vi "Multiserver Example.vi"() -> ()   [LabVIEW 2013]
uses:
  LabVIEW Core/Ports - Keep-Alive, LabVIEW-to-Python, Python-to-LabVIEW.ctl
  LabVIEW Core/TS.lvlib
panel:
  in  "Local IP Address for LabVIEW Server 2":string="localhost"
  in  "Ports 2":T1={"KA Port (9007)"=9010, "LtoP Port (9008)"=9011, "PtoL Port (9009)"=9012}
  in  "Server Alias 2":string="Test Group 2"
  in  "Local IP Address for LabVIEW Server 1":string="localhost"
  in  "Ports 1":T1={"KA Port (9007)"=9007, "LtoP Port (9008)"=9008, "PtoL Port (9009)"=9009}
  in  "Server Alias 1":string="Test Group 1"
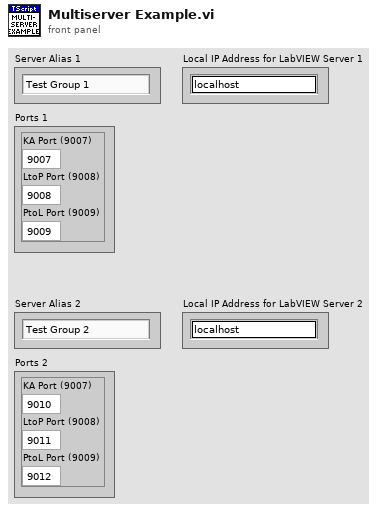
[diagram p1: front panel]
types:
  T1 = typedef "TS.lvlib/Ports - Keep-Alive, LabVIEW-to-Python, Python-to-LabVIEW.ctl" = cluster{"KA Port (9007)":u16, "LtoP Port (9008)":u16, "PtoL Port (9009)":u16}
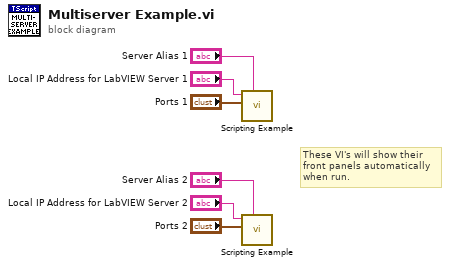
[diagram p0: block diagram]
diagram:
  # "These VI's will show their\nfront panels automatically \nwhen run."
  n1 = call "Scripting Example.vi"("Server Alias"="Server Alias 1", "Ports"="Ports 1", "Local IP Address for LabVIEW Server"="Local IP Address for LabVIEW Server 1") -> ()  [unwired: 9 in]
  n2 = call "Scripting Example.vi"("Server Alias"="Server Alias 2", "Ports"="Ports 2", "Local IP Address for LabVIEW Server"="Local IP Address for LabVIEW Server 2") -> ()  [unwired: 9 in]
